vi "Find Module Specific Config.vi"(10 "Module ID":string, 11 "Standard Engine Repo Data in":refnum<class "Standard Engine Configuration.lvclass">) -> (2 "Index":i32, 3 "Standard Engine Repo Data out":refnum<class "Standard Engine Configuration.lvclass">)   [LabVIEW 2013, in "Standard Engine Configuration.lvclass"]
uses:
  Standard Engine Configuration.lvclass
  Standard Engine Configuration.lvclass/Standard Engine Configuration.ctl
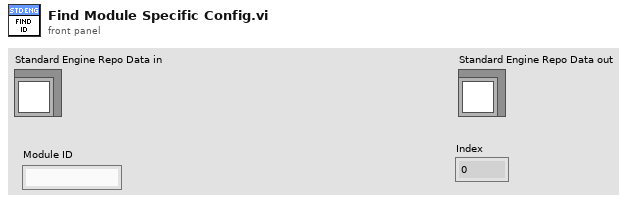
[diagram p1: front panel]
types:
  T1 = typedef "Standard Engine Configuration.lvclass/Module Specific Configuration.ctl" = cluster{"Module ID":string, "Module Decimation":T2, "error tag":string, "error responses":T3}
  T2 = typedef "Standard Engine Configuration.lvclass/Module Decimation.ctl" = cluster{"Decimation":u16, "Offset":u16, "sort order":i32, "async?":bool}
  T3 = typedef "Standard Engine Configuration.lvclass/error responses.ctl" = cluster{"unknown":T4, "trivial":T4, "critical":T4, "recoverable":T4}
  T4 = typedef "Standard Engine Configuration.lvclass/error options.ctl" = cluster{"clear":bool, "notify":bool, "log":bool, "remove module":bool, "abort engine":bool, "go to safe state":bool, "recover module":bool}
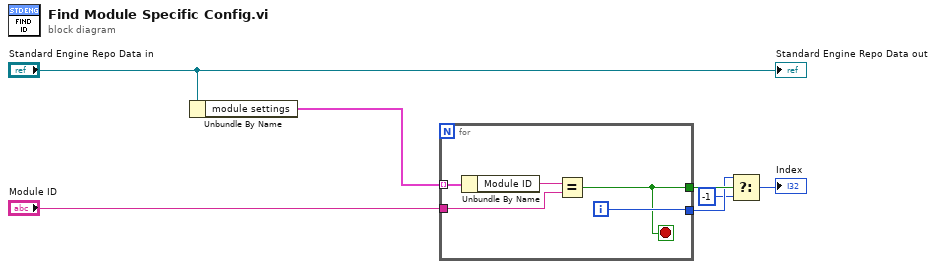
[diagram p0: block diagram]
diagram:
  n1 = Unbundle By Name("Standard Engine Repo Data in") -> ("module settings"=w5:T1[])
  n2 = for {
    tunnel: "Module ID" -> [w10]
    tunnel: w5 -> [w12] mode=indexing
    tunnel: [w9] -> w3
    tunnel: [w8] -> w4
    i -> [w9]
    stop <- w8 stop-if-true
    n3 = Unbundle By Name(w12) -> ("Module ID"=w11:string)
    n4 = Equal?(x=w11, y=w10) -> (x = y?=w8:bool)
  }
  n5 = Select(t=w3, s=w4, f=-1) -> (s? t:f=→"Index":i32)
  "Standard Engine Repo Data out" <- "Standard Engine Repo Data in"
